vi "FlexDDS-NG_DCP_WriteSTP.vi"(4 "phase degrees (0..360)":dbl, 6 "amplitude (0..1)":dbl=1.0, 7 "mirror frequency?":bool, 8 "frequency Hz (0..400M)":dbl=10000000.0 format="%^#_6e", 9 "single tone profile (0..7)":i32 min=0 max=7 step=1, 10 "Channels":T1(ring)=enum."Both channels", 11 "initial instruction string":string) -> (3 "appended instruction string":string)   [LabVIEW 2016]
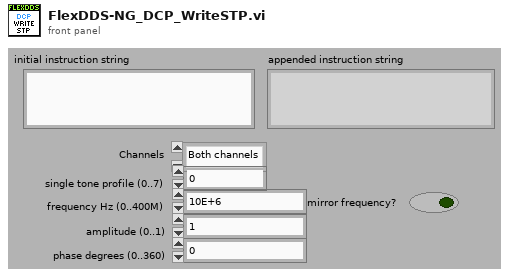
[diagram p1: front panel]
types:
  T1 = enum32{"Channel 0", "Channel 1", "Both channels"}
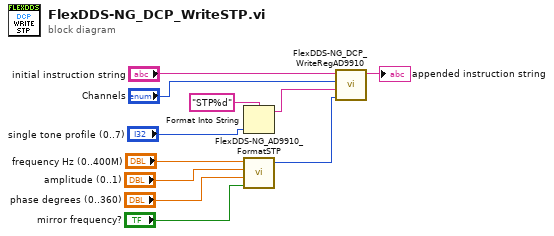
[diagram p0: block diagram]
diagram:
  n1 = Format Into String(format string="STP%d", "single tone profile (0..7)") -> (resulting string=w6:string)  [unwired: 2 in, 1 out]
  n2 = call "FlexDDS-NG_AD9910_FormatSTP.vi"("mirror frequency?"="mirror frequency?", "phase degrees (0..360)"="phase degrees (0..360)", "amplitude (0..1)"="amplitude (0..1)", "Frequency Hz (0)"="frequency Hz (0..400M)") -> ("single-tone profile (STP) out"=w5:u64)  [unwired: 4 in, 3 out]
  n3 = call "FlexDDS-NG_DCP_WriteRegAD9910.vi"("register content"=w5, "AD9910 register name"=w6, "Channels"="Channels", "initial instruction string"="initial instruction string") -> ("appended instruction string"=→"appended instruction string":string)  [unwired: 7 in]
